vi "M_Config232Port.vi"(1 "timeout (ms)":u32=10000, 2 "error in (no error)":errorcluster {"code" format="%.0x"}, 3 "baud rate":u32=9600, 4 "Enum":enum16{"Init ComPort", "UnInit ComPort"}(ring), 5 "VISA resource name":refnum<visa-resource-name>="COM1") -> (0 "error out":errorcluster)   [LabVIEW 2014]
uses:
  <vilib>/Instr/_visa.llb/VISA Set IO Buffer Mask.ctl
  <vilib>/Instr/_visa.llb/VISA Configure Serial Port (Instr).vi
panel:
  in  "termination char (0xA = '\\n' = LF)":u8=10 format="%.0x"
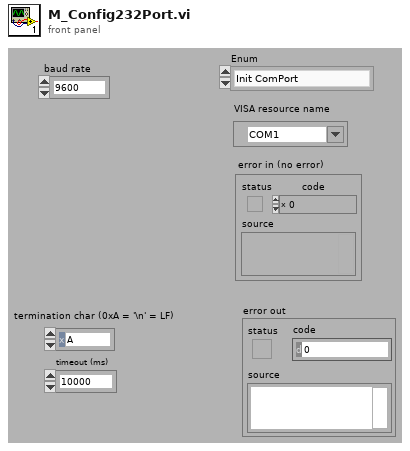
[diagram p1: front panel]
types:
  T1 = typedef "VISA Set IO Buffer Mask.ctl" = u16
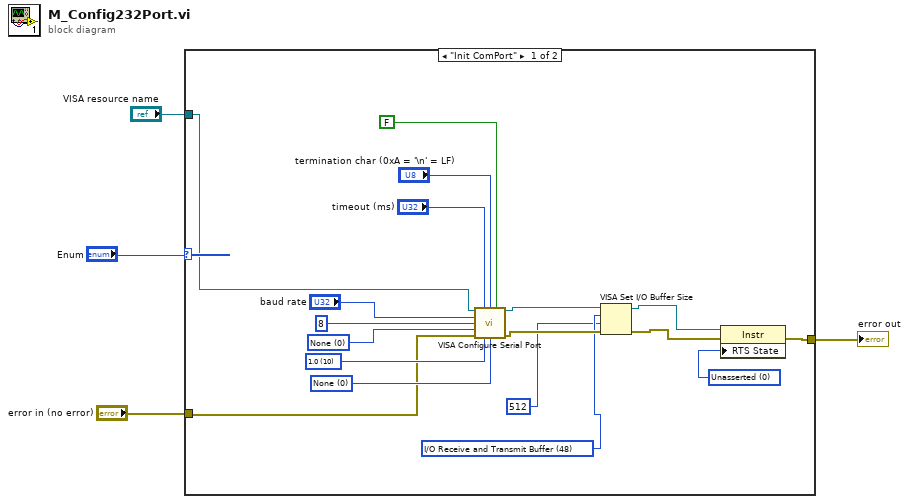
[diagram p0: block diagram]
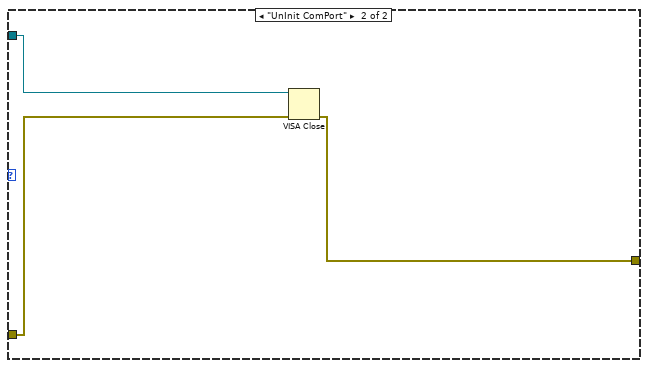
[diagram p2: hidden frame]
diagram:
  n1 = case shown="\"Init ComPort\"" "Enum" {
    tunnel: "VISA resource name" -> [w14 w25]
    tunnel: "error in (no error)" -> [w13 w24]
    tunnel: [w12 w23] -> w2
    frame "Init ComPort" {
      w8 = T1 48 items=["I/O Receive Buffer"=16, "I/O Transmit Buffer"=32, "I/O Receive and Transmit Buffer"=48] ("Mask")
      w17 = u16 0 items=["None"=0, "XON/XOFF"=1, "RTS/CTS"=2, "DTR/DSR"=4] ("flow control")
      w20 = u16 10 items=["1.0"=10, "1.5"=15, "2.0"=20] ("stop bits")
      w21 = u16 0 items=["None", "Odd", "Even", "Mark", "Space"] ("parity")
      w11 = i16 0 items=["Unknown"=-1, "Unasserted"=0, "Asserted"=1] ("Serial Settings:Modem Line Settings:Line RTS State")
      n2 = call-poly "VISA Configure Serial Port"("VISA resource name"=w14, "timeout (10sec)"="timeout (ms)", "termination char\n(0xA = '\\n' = LF)"="termination char (0xA = '\\n' = LF)", "Enable Termination\nChar (T)"=FALSE ("End read on termination character? 2"), "baud rate (9600)"="baud rate", "data bits (8)"=u16 8 ("data bits"), "parity (0:none)"=w21, "error in (no error)"=w13, "stop bits (10: 1 bit)"=w20, "flow control (0:none)"=w17) -> ("VISA resource name out"=w9:refnum<visa-resource-name>, "error out"=w10:errorcluster)  [unwired: 4 in]
      n3 = VISA Set I/O Buffer Size(VISA resource name=w9, mask (16)=w8, size (4096)=u32 512, error in (no error)=w10) -> (VISA resource name out=w6:refnum<visa-resource-name>, error out=w5:errorcluster)
      n4 = property class="Instr"(reference=w6, error in=w5, "RTS State"=w11) -> (error out=w12:errorcluster)  [unwired: 1 out]
    }
    frame "UnInit ComPort" {
      n5 = VISA Close(VISA resource name=w25, error in (no error)=w24) -> (error out=w23:errorcluster)
    }
  }
  "error out" <- w2
